vi "EnqueueMessage(Single).vi"(6 "Priority Message? (F)":bool, 8 "error in (no error)":errorcluster, 9 "Message Data":variant, 10 "Message":string, 11 "Message Queue":refnum<queue>) -> (0 "error out":errorcluster, 3 "dup Message Queue":refnum<queue>)   [LabVIEW 2017, in "Server.lvlib" / "Message Queue.lvlib"]
doc: "For a regular message, enqueue the message. For a priority message, enqueue it at the front of the queue."
uses:
  Message Queue.lvlib
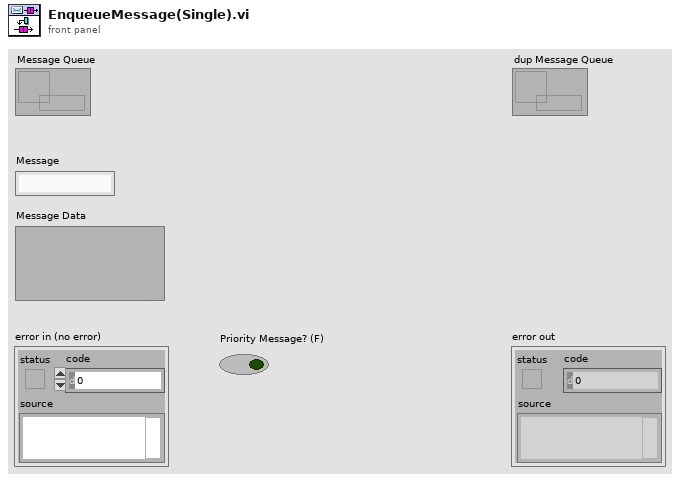
[diagram p1: front panel]
types:
  T1 = cluster{"Message":string, "Message Data":variant}
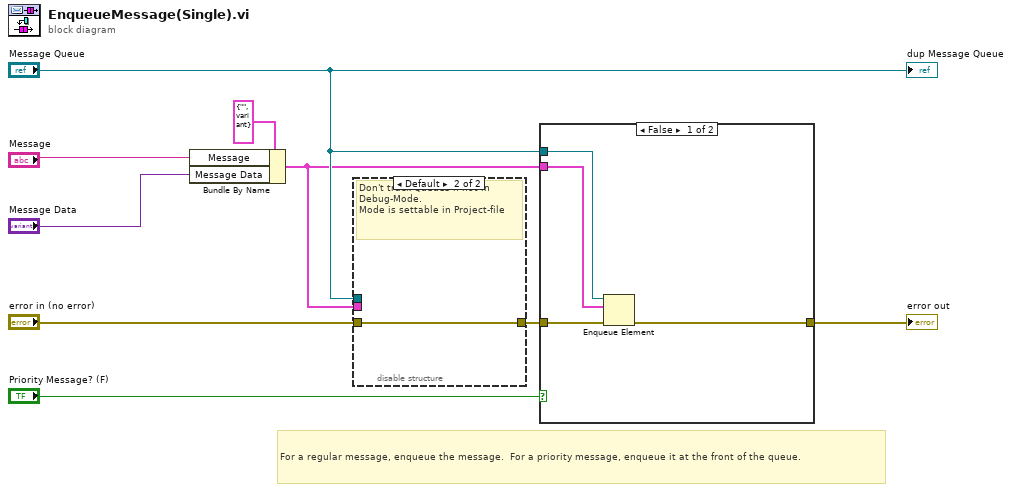
[diagram p0: block diagram]
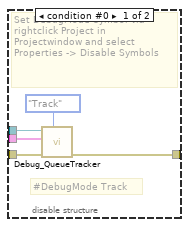
[diagram p2: hidden frame]
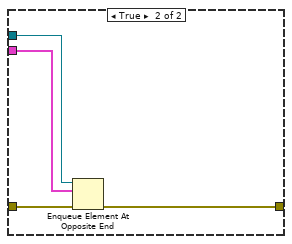
[diagram p3: hidden frame]
diagram:
  # "For a regular message, enqueue the message.  For a priority message, enqueue it at the front of the queue."
  n1 = Bundle By Name(cluster=T1 {"Message"="", "Message Data"=variant} ("Message Cluster"), "Message"="Message", "Message Data"="Message Data") -> (w1:T1)
  n2 = disable-structure shown="Default" {
    disable-tunnel: "error in (no error)" -> [w14 w15]
    disable-tunnel: [w13 w15] -> w3
    disable-tunnel: "Message Queue" -> [w12 _]
    disable-tunnel: w1 -> [w11 _]
    frame condition #0 {
      # "#DebugMode Track"
      # "Set DebugMode-Symbol via\nrightclick Project in Projectwindow and select Properties -> Disable Symbols"
      n3 = call "Debug_QueueTracker.vi"("Mode"=enum16{"Init", "Track", "DeInit"}."Track", "Error In"=w14, "Message Cluster"=w11, "QueueIn"=w12) -> ("Error Out"=w13:errorcluster)  [unwired: 7 in]
    }
    frame condition #1 (active) {
      # "Don't track Queues if not in \nDebug-Mode.\nMode is settable in Project-file"
    }
  }
  n4 = case shown="False" "Priority Message? (F)" {
    tunnel: w3 -> [w19 w23]
    tunnel: [w18 w22] -> w4
    tunnel: "Message Queue" -> [w17 w21]
    tunnel: w1 -> [w16 w20]
    frame False {
      n5 = Enqueue Element(queue=w17, element=w16, error in (no error)=w19) -> (error out=w18:errorcluster)  [unwired: 1 in, 2 out]
    }
    frame True {
      n6 = Enqueue Element At Opposite End(queue=w21, element=w20, error in (no error)=w23) -> (error out=w22:errorcluster)  [unwired: 1 in, 2 out]
    }
  }
  "error out" <- w4
  "dup Message Queue" <- "Message Queue"
